vi "Logging_PathConfig.vi"(8 "Seed2":i32, 9 "Seed1":i32, 10 "Excitation Duration":i32, 11 "Period":i32) -> (1 "Data path 2":path, 2 "Model path":path)   [LabVIEW 2015]
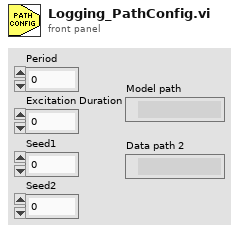
[diagram p1: front panel]
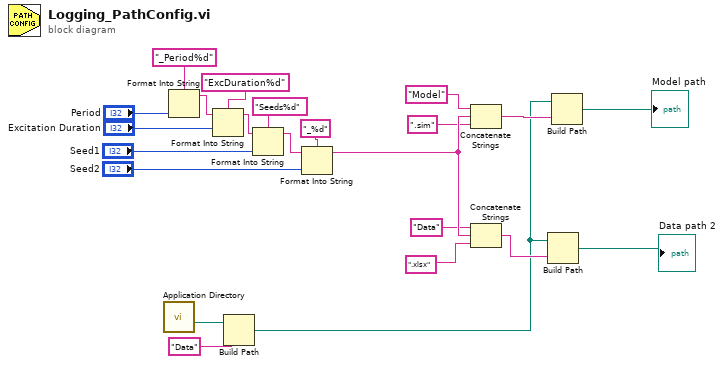
[diagram p0: block diagram]
diagram:
  n1 = call <vilib>:"Application Directory.vi"() -> ("Application Directory"=w14:path)
  n2 = Format Into String(format string="_Period%d", "Period") -> (resulting string=w7:string)  [unwired: 2 in, 1 out]
  n3 = Format Into String(format string="ExcDuration%d", initial string=w7, "Excitation Duration") -> (resulting string=w8:string)  [unwired: 1 in, 1 out]
  n4 = Build Path(base path=w14, name or relative path="Data") -> (appended path=w5:path)
  n5 = Format Into String(format string="Seeds%d", initial string=w8, "Seed1") -> (resulting string=w9:string)  [unwired: 1 in, 1 out]
  n6 = Format Into String(format string="_%d", initial string=w9, "Seed2") -> (resulting string=w21:string)  [unwired: 1 in, 1 out]
  n7 = Concatenate Strings("Model" ("string"), w21, ".sim" ("string")) -> (w22:string)
  n8 = Concatenate Strings("Data" ("string"), w21, ".xlsx" ("string")) -> (w16:string)
  n9 = Build Path(base path=w5, name or relative path=w16) -> (appended path=→"Data path 2":path)
  n10 = Build Path(base path=w5, name or relative path=w22) -> (appended path=→"Model path":path)
